vi "Notificador.vi"() -> ()   [LabVIEW 2016]
uses:
  <extravilib>/ChannelInstances/Stream-dbl/Read With Abort.vi
  <extravilib>/ChannelInstances/Stream-dbl/Write With Abort.vi
  <extravilib>/ChannelInstances/Stream-dbl/Endpoint.vi
  <extravilib>/ChannelInstances/Stream-dbl/Instantiate.vi
  <extravilib>/ChannelInstances/Stream-dbl/)Channel.vi
  <resource>/ChannelSupport/_ChannelSupport/WaitIfNeeded.vi
  <extravilib>/ChannelInstances/Stream-dbl.lvlib
panel:
  out "sin(x) 2":dbl(graph)
  in  "Stop Button 2":bool
  in  "milliseconds to wait 2":u32=15
  out "Numeric Control 2":i32
  out "Numeric Control":i32
  in  "milliseconds to wait":u32=15
  in  "Stop Button":bool
  out "sin(x)":dbl(graph)
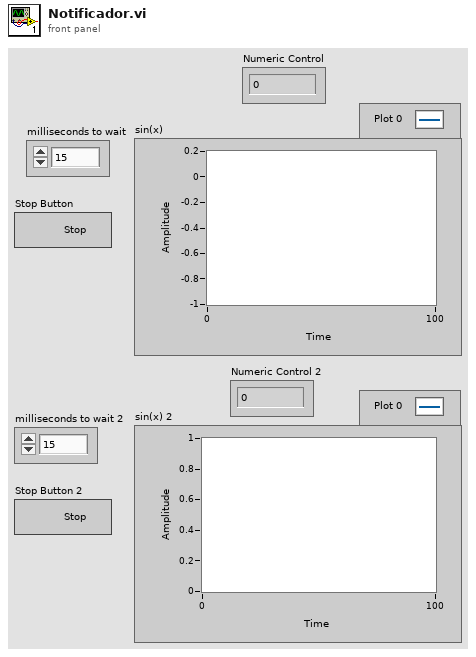
[diagram p1: front panel]
types:
  T1 = typedef "Stream-dbl.lvlib/)Channel.ctl" = refnum<queue>
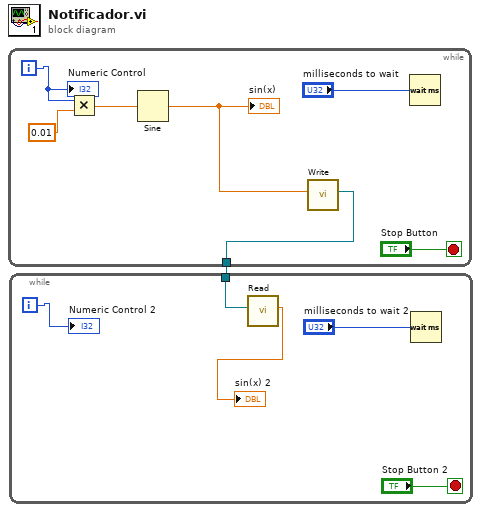
[diagram p0: block diagram]
diagram:
  n1 = while {
    tunnel: [w2] -> w1
    i -> [w8]
    stop <- "Stop Button" stop-if-true
    n2 = Multiply(x=w8, y=0.01) -> (x*y=w6:dbl)
    n3 = Sine(x=w6) -> (sin(x)=w3:dbl)
    "sin(x)" <- w3
    n4 = call <extravilib>:"Write.vi"("element"=w3) -> ("channel"=w2:T1)  [unwired: 8 in, 2 out]
    n5 = Wait (ms)(milliseconds to wait="milliseconds to wait") -> ()  [unwired: 1 out]
    "Numeric Control" <- w8
  }
  n6 = while {
    tunnel: w1 -> [w10]
    i -> [w13]
    stop <- "Stop Button 2" stop-if-true
    n7 = call <extravilib>:"Read.vi"("channel"=w10) -> ("element"=→"sin(x) 2":dbl)  [unwired: 6 in, 4 out]
    n8 = Wait (ms)(milliseconds to wait="milliseconds to wait 2") -> ()  [unwired: 1 out]
    "Numeric Control 2" <- w13
  }
